vi "Get Model Serial (SubVI).vi"(0 "CmdLib In":refnum<k24>, 5 "DeviceKey In":string, 9 "Device Address In":i32, 11 "error in (no error)":errorcluster) -> (4 "CmdLib Out":refnum<k24>, 6 "DeviceKey Out":string, 8 "Device Address Out":i32, 10 "Model / Serial":string, 15 "error out":errorcluster)   [LabVIEW 2017]
uses:
  dll/CmdLib.dll
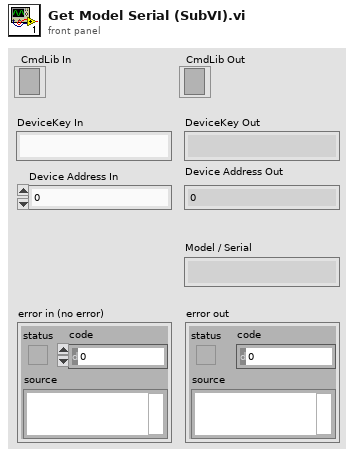
[diagram p1: front panel]
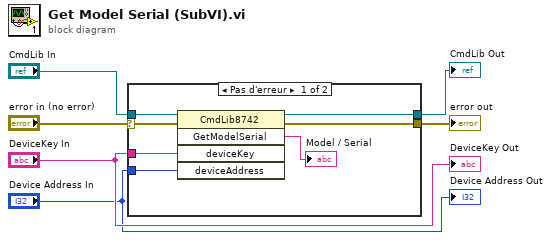
[diagram p0: block diagram]
diagram:
  n1 = case shown="Pas d'erreur" "error in (no error)" {
    selector: "error in (no error)" -> [w10 w15]
    tunnel: "CmdLib In" -> [w13 w14]
    tunnel: [w12 w14] -> w5
    tunnel: "DeviceKey In" -> [w11 _]
    tunnel: [w9 w15] -> w2
    tunnel: "Device Address In" -> [w7 _]
    frame No Error {
      n2 = invoke class="CmdLib8742" method="GetModelSerial"(reference=w13, error in=w10, "deviceKey"=w11, "deviceAddress"=w7) -> (reference out=w12:refnum<k24>, error out=w9:errorcluster, "GetModelSerial"=→"Model / Serial":string)  [unwired: 1 in, 2 out]
    }
    frame Error {
    }
  }
  "CmdLib Out" <- w5
  "error out" <- w2
  "DeviceKey Out" <- "DeviceKey In"
  "Device Address Out" <- "Device Address In"
